vi "Load script file.vi"() -> (1 "Array":T1[](array[typedef]) {"Carousel" items=["0", "1", "2", "3", "4", "5", "6"]; "Angle [°]" min=0.0 max=350.0; "Tau [ms]" min=0.0 max=100.0; "Wait [min]" min=0.0 max=350.0; "Tmp [K]" min=0.0 max=3000.0; "Mod_A [G]" min=0.1 max=150.0; "Mod_F [kHz]" min=0.1 max=150.0}, 2 "Multiplication factor":i32)   [LabVIEW 2024]
uses:
  Datatypes/script polymorh line.ctl
  <vilib>/Utility/config.llb/Read Key (I32).vi
  <vilib>/Utility/config.llb/NI_LVConfig.lvlib
  <userlib>/_OpenG.lib/variantconfig/variantconfig.llb/openg_variant_configuration_file.lvlib
panel:
  in  "error in":errorcluster
  out "error out":errorcluster
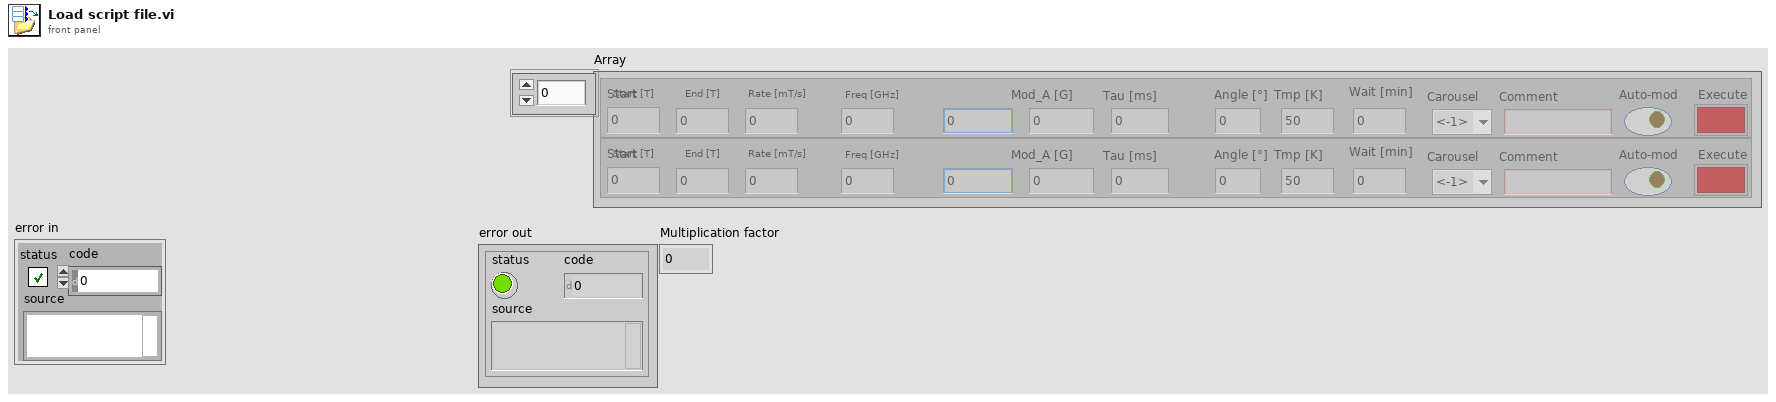
[diagram p1: front panel]
types:
  T1 = typedef "script polymorh line.ctl" = cluster{"Start":dbl, "Start Caption":string, "End":dbl, "End Caption":string, "Sweep":dbl, "Sweep caption":string, "Constant":dbl, "Constant caption":string, "Mod_F [kHz]":dbl, "Mod_A [G]":dbl, "Tau [ms]":dbl, "Angle [°]":dbl, "Tmp [K]":dbl, "Wait [min]":dbl, "Carousel":i8, "Comment":string, "Auto-mod":bool, "Execute":bool}
  T2 = typedef "NI_LVConfig.lvlib/Config Data RefNum.ctl" = refnum<k1>
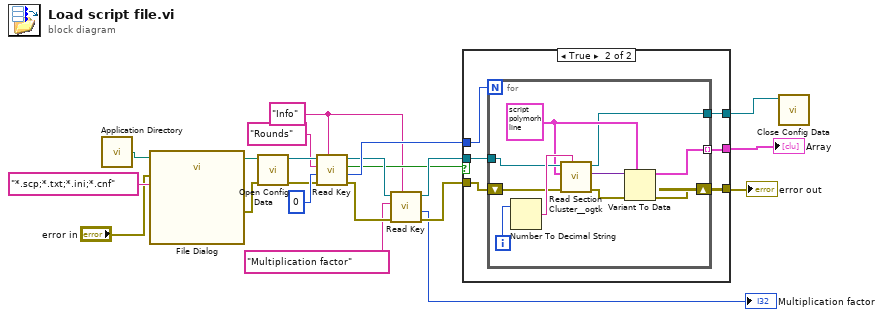
[diagram p0: block diagram]
diagram:
  w7 = "Info" ("section")
  n1 = call <vilib>:"Application Directory.vi"() -> ("Application Directory"=w15:path)
  n2 = call "File Dialog"("start path"=w15, "error in"="error in", "pattern (all files)"="*.scp;*.txt;*.ini;*.cnf" ("string")) -> ("selected path"=w13:path, "error out"=w14:errorcluster)  [unwired: 9 in, 2 out]
  n3 = call <vilib>:"Open Config Data.vi"("error in (no error)"=w14, "configuration file path"=w13) -> ("error out"=w19:errorcluster, "refnum"=w18:T2)  [unwired: 7 in, 1 out]
  n4 = call-poly <vilib>:"Read Key.vi"("section"=w7, "error in (no error)"=w19, "default value"=0, "key"="Rounds", "refnum"=w18) -> ("error out"=w6:errorcluster, "value"=w21:i32, "found?"=w8:bool, "refnum out"=w10:T2)  [unwired: 3 in]
  n5 = call-poly <vilib>:"Read Key.vi"("section"=w7, "error in (no error)"=w6, "key"="Multiplication factor", "refnum"=w10) -> ("error out"=w4:errorcluster, "value"=→"Multiplication factor":i32, "refnum out"=w9:T2)  [unwired: 4 in, 1 out]
  n6 = case shown="True" w8 {
    tunnel: w9 -> [w22 w29]
    tunnel: w21 -> [_ w28]
    tunnel: w4 -> [w23 w27]
    tunnel: [_ w26] -> w1
    tunnel: [w23 w25] -> w12
    tunnel: [w22 w24] -> w2
    frame False {
    }
    frame True {
      n7 = for {
        N: w28 -> [_]
        tunnel: w29 -> [w37]
        shift-right: [w34] -> w25
        shift-left: w27 -> [w36]
        tunnel: [w31] -> w26 mode=indexing
        tunnel: [w30] -> w24
        i -> [w39]
        w32 = T1 {"Start"=0.0, "Start Caption"="Start [T]", "End"=0.0, "End Caption"="End [T]", "Sweep"=0.0, "Sweep caption"="Rate [mT/s]", "Constant"=0.0, "Constant caption"="Freq [GHz]", "Mod_F [kHz]"=0.0, "Mod_A [G]"=0.0, "Tau [ms]"=0.0, "Angle [°]"=0.0, "Tmp [K]"=50.0, "Wait [min]"=0.0, "Carousel"=-1, "Comment"="", "Auto-mod"=TRUE, "Execute"=FALSE} ("Row")
        n8 = Number To Decimal String(number=w39) -> (decimal integer string=w38:string)  [unwired: 1 in]
        n9 = call <userlib>:"Read Section Cluster__ogtk.vi"("section (optional)"=w38, "error in (no error)"=w36, "Section Formatted Cluster Type"=w32, "refnum"=w37) -> ("error out"=w33:errorcluster, "Section Formatted Cluster"=w35:variant, "dup refnum"=w30:T2)  [unwired: 3 in, 2 out]
        n10 = Variant To Data(error in=w33, type=w32, Variant=w35) -> (data=w31:T1, error out=w34:errorcluster)
      }
    }
  }
  "error out" <- w12
  "Array" <- w1
  n11 = call <vilib>:"Close Config Data.vi"("refnum"=w2) -> ()  [unwired: 9 in, 2 out]
